vi "Iterations_Until_Integar_Equals.vi"() -> ()   [LabVIEW 2022 SP3]
uses:
  <vilib>/numeric/Random Number (Range) I64.vi
  <vilib>/numeric/sub_Random U32.vi
panel:
  in  "Max":i32=100
  out "Number of Iterations":i32
  in  "Target Number":dbl
  # "Iterations_Until_Integar_Equals:\nBegin by selecting an upper bound for the random number.\nThen select a target number.\nThe number of iterations until the random number matches\nthe target number is displayed."
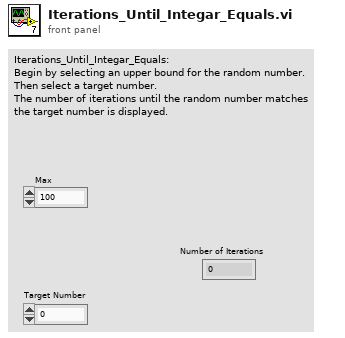
[diagram p1: front panel]
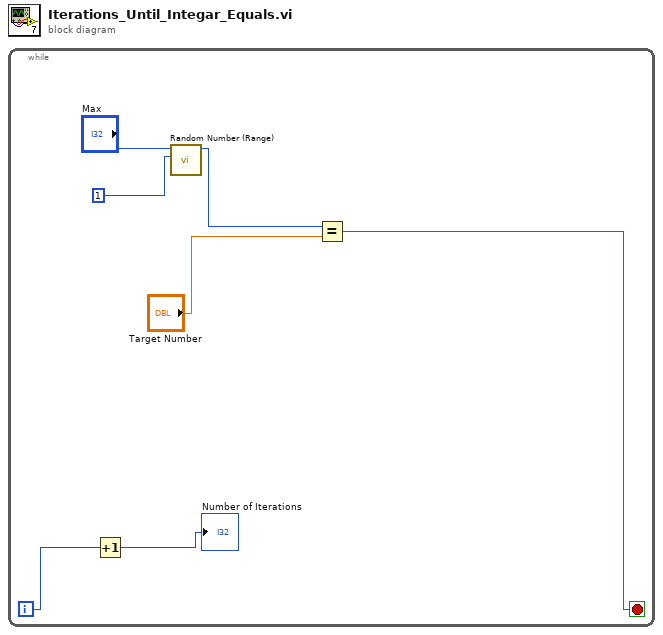
[diagram p0: block diagram]
diagram:
  n1 = while {
    i -> [w2]
    stop <- w3 stop-if-true
    n2 = Increment(x=w2) -> (x+1=→"Number of Iterations":i32)
    n3 = call-poly <vilib>:"Random Number (Range).vi"("lower bound (-100)"=1, "upper bound (100)"="Max") -> ("number"=w5:i64)  [unwired: 9 in]
    n4 = Equal?(x=w5, y="Target Number") -> (x = y?=w3:bool)
  }
